vi "Set Digital Out.vi"(8 "error in":errorcluster, 11 "MiniIO in":refnum<class "MiniIO.lvclass">) -> (0 "error out":errorcluster, 3 "MiniIO out":refnum<class "MiniIO.lvclass">)   [LabVIEW 2018, in "MiniIO.lvlib" / "MiniIO.lvclass"]
uses:
  MiniIO.lvclass
  PPLs/PLC/Parent/PLC.lvlibp/PLC.lvclass
  C:/AME Test Engineering/LabVIEW/PPLs/PLC/Parent/PLC.lvlibp/PLC.lvclass
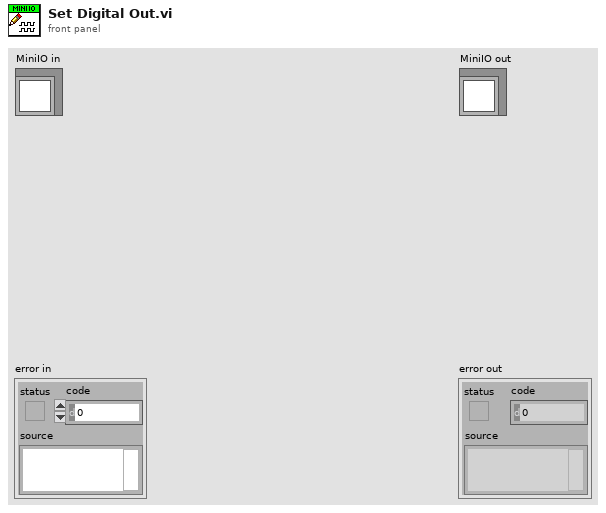
[diagram p1: front panel]
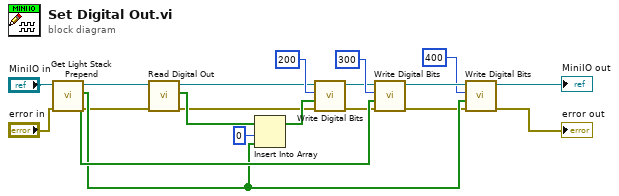
[diagram p0: block diagram]
diagram:
  n1 = call "Get Light Stack Prepend.vi"("error in"="error in", "MiniIO in"="MiniIO in") -> ("error out"=w1:errorcluster, "Blink Memory"=w16:bool[], "D/O Prepend"=w13:bool[], "MiniIO out"=w2:refnum<class "MiniIO.lvclass">)  [unwired: 6 in]
  n2 = call "Read Digital Out.vi"("error in"=w1, "PLC in"=w2) -> ("error out"=w3:errorcluster, "Digital Out"=w4:bool[], "PLC out"=w5:refnum<class "MiniIO.lvclass">)  [unwired: 7 in]
  n3 = Insert Into Array(array=w4, index=0, new element=w13) -> (w15:bool[])
  n4 = call "Write Digital Bits.vi"("error in"=w3, "Bits:"=w15, "Memory Start:"=u16 200, "MiniIO in"=w5) -> ("error out"=w9:errorcluster, "MiniIO out"=w10:refnum<class "MiniIO.lvclass">)  [unwired: 6 in]
  n5 = call "Write Digital Bits.vi"("error in"=w9, "Bits:"=w16, "Memory Start:"=u16 300, "MiniIO in"=w10) -> ("error out"=w7:errorcluster, "MiniIO out"=w8:refnum<class "MiniIO.lvclass">)  [unwired: 6 in]
  n6 = call "Write Digital Bits.vi"("error in"=w7, "Bits:"=w13, "Memory Start:"=u16 400, "MiniIO in"=w8) -> ("error out"=→"error out":errorcluster, "MiniIO out"=→"MiniIO out":refnum<class "MiniIO.lvclass">)  [unwired: 6 in]
